vi "setModbusRxDataFIFO.vi"(10 "ModbusRxDataFIFO":refnum<class "IReadU16FIFO.lvclass">, 11 "ILCCommunications in":refnum<class "ILCCommunications.lvclass">) -> (3 "ILCCommunications out":refnum<class "ILCCommunications.lvclass">)   [LabVIEW 2016, in "ILCCommunications.lvclass"]
uses:
  ILCCommunications.lvclass
  Common_RT_FPGA/IReadU16FIFO/IReadU16FIFO.lvclass
  ILCCommunications.lvclass/ILCCommunications.ctl
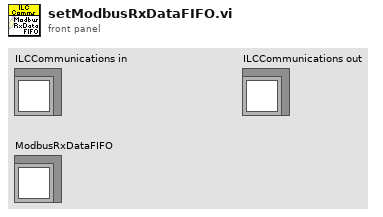
[diagram p1: front panel]
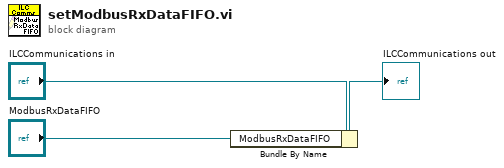
[diagram p0: block diagram]
diagram:
  n1 = Bundle By Name(cluster="ILCCommunications in", "ModbusRxDataFIFO"="ModbusRxDataFIFO") -> (→"ILCCommunications out":refnum<class "ILCCommunications.lvclass">)
